vi "Change Tag Output.vi"(6 "Variant":variant, 8 "error in":errorcluster, 9 "old values":string[][](array[string]), 10 "object ref in":T1, 11 "Cluster":T2) -> (0 "error out":errorcluster)   [LabVIEW 2013, in "Shared Memory Editor Node.lvclass"]
doc: "Copyright 2016 National Instruments Corporation\n\nLicensed under the Apache License, Version 2.0 (the \"License\"); you may not use this file except in compliance with the License. You may obtain a copy of the License at http://www.apache.org/licenses/LICENSE-2.0\nUnless required by applicable law or agreed to in writing, software distributed under the License is distributed on an \"AS IS\" BASIS, WITHOUT WARRANTIES OR CONDITIONS OF ANY KIND, either express or implied. See the License for the specific language governing permissions and limitations under the License."
uses:
  Shared Memory Editor Node.lvclass
  <vilib>/NI/DCAF Table API/Table Manager/Cell Change.ctl
  <vilib>/NI/DCAF Table API/Table Manager/object ref.ctl
  <vilib>/NI/DCAF/Tag Editor Core/Configuration Editor/Classes/Engine Parent/Engine Parent Editor Node.lvclass
  <vilib>/NI/DCAF/Tag Editor Core/Configuration Editor/Classes/Module editor node/module editor node.lvclass
  <vilib>/NI/Tag Bus Module Framework/channel/TBM channel.lvclass
  <vilib>/NI/Tag Bus/tag/tag descriptor.lvclass/tag descriptor.ctl
  module/configuration/Shared Memory Configuration.lvclass
  module/configuration/Shared Memory Configuration.lvclass/Shared Memory Configuration.ctl
  <vilib>/NI/Tag Bus/tag/tag descriptor.lvclass
  <vilib>/NI/DCAF Table API/Table Manager.lvlib
  <vilib>/NI/DCAF Table API/Table Manager/Table Manager.lvclass
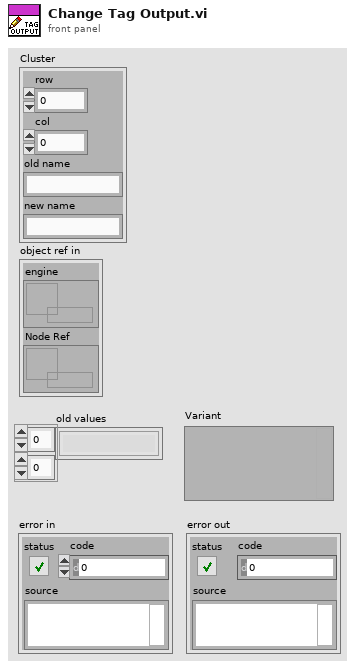
[diagram p1: front panel]
types:
  T1 = typedef "Table Manager.lvlib/Table Manager.lvclass/object ref.ctl" = cluster{"engine":refnum<data-value>, "Node Ref":refnum<data-value>}
  T2 = typedef "Table Manager.lvlib/Cell Change.ctl" = cluster{"row":i32, "col":i32, "old name":string, "new name":string}
  T3 = typedef "Shared Memory Configuration.lvclass/line configuration.ctl" = cluster{"name":string, "data type":T4, "channel":refnum<class "TBM channel.lvclass">}
  T4 = typedef "tag bus.lvlib/tag descriptor.lvclass/Data Type.ctl" = enum16{"Double", "Single", "I64", "I32", "I16", "I8", "U64", "U32", "U16", "U8", "Boolean", "String", "Array of Double", "Array of Single", "Array of I64", "Array of I32", "Array of I16", "Array of I8", "Array of U64", "Array of U32", "Array of U16", "Array of U8", "Array of Boolean", "Array of String"}
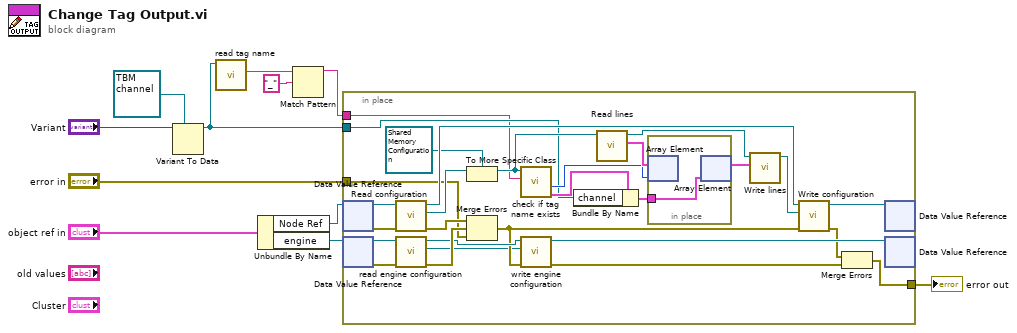
[diagram p0: block diagram]
diagram:
  n1 = Variant To Data(type=refnum<class "TBM channel.lvclass"> refnum ("output"), Variant="Variant") -> (data=w4:refnum<class "TBM channel.lvclass">)  [unwired: 1 in, 1 out]
  n2 = call <vilib>:"read tag name.vi"("system tag in"=w4) -> ("name"=w3:string)  [unwired: 8 in, 2 out]
  n3 = Unbundle By Name("object ref in") -> ("Node Ref"=w7:refnum<data-value>, "engine"=w6:refnum<data-value>)
  n4 = Match Pattern(string=w3, regular expression="_") -> (before substring=w1:string)  [unwired: 1 in, 3 out]
  n5 = in-place {
    in-place-border: [w31] -> w11
    in-place-border: "error in" -> [w23]
    in-place-border: w4 -> [w14]
    in-place-border: w1 -> [w13]
    n6 = in-place-dvr #1(w7) -> (w28:refnum<class "module editor node.lvclass">, w30:errorcluster)
    n7 = in-place-dvr #2(w6) -> (w38:refnum<class "Engine Parent Editor Node.lvclass">, w39:errorcluster)
    n8 = call-dynamic "Read configuration.vi"("error in"=w30, "NISE_CEF_serializable node in"=w28) -> ("error out"=w29:errorcluster, "configuration"=w26:refnum<class "NISE_CEF_serializable configuration.lvclass">, "NISE_CEF_serializable node out"=w27:refnum<class "module editor node.lvclass">)  [unwired: 7 in]
    n9 = call <vilib>:"read engine configuration.vi"("error in"=w39, "Engine Parent Editor Node in"=w38) -> ("error out"=w35:errorcluster, "engine configuration"=w12:refnum<class "engine configuration.lvclass">, "Engine Parent Editor Node out"=w34:refnum<class "Engine Parent Editor Node.lvclass">)  [unwired: 7 in]
    n10 = To More Specific Class(target class=refnum<class "Shared Memory Configuration.lvclass"> refnum ("tag select module configuration"), reference=w26) -> (specific class reference=w22:refnum<class "Shared Memory Configuration.lvclass">)  [unwired: 1 in, 1 out]
    n11 = Merge Errors(w29, w35, w23) -> (w25:errorcluster)
    n12 = call "check if tag name exists.vi"("name to locate"=w13, "shared memory module configuration in"=w22) -> ("tag config"=w17:T3, "index"=w18:i32)  [unwired: 6 in, 2 out]
    n13 = call <vilib>:"write engine configuration.vi"("error in"=w25, "engine configuration"=w12, "Engine Parent Editor Node in"=w34) -> ("error out"=w33:errorcluster, "Engine Parent Editor Node out"=w37:refnum<class "Engine Parent Editor Node.lvclass">)  [unwired: 7 in]
    n14 = Bundle By Name(cluster=w17, "channel"=w14) -> (w16:T3)
    n15 = call "Read lines.vi"("shared memory module configuration"=w22) -> ("lines"=w21:T3[], "shared memory module configuration out"=w19:refnum<class "Shared Memory Configuration.lvclass">)  [unwired: 8 in, 1 out]
    n16 = in-place {
      in-place-border: w16 -> [w40]
      n17 = in-place-array #3(w21, w18) -> ()  [unwired: 1 out]
      n18 = in-place-array #3(w40) -> (w20:T3[])  [unwired: 1 out]
    }
    n19 = call "Write lines.vi"("lines"=w20, "shared memory module configuration"=w19) -> ("shared memory module configuration out"=w15:refnum<class "Shared Memory Configuration.lvclass">)  [unwired: 8 in, 1 out]
    n20 = call-dynamic "Write configuration.vi"("error in"=w25, "configuration"=w15, "NISE_CEF_serializable node in"=w27) -> ("error out"=w32:errorcluster, "NISE_CEF_serializable node out"=w36:refnum<class "module editor node.lvclass">)  [unwired: 7 in]
    n21 = Merge Errors(w32, w33) -> (w31:errorcluster)
    n22 = in-place-dvr #1(w36) -> ()  [unwired: 2 out]
    n23 = in-place-dvr #2(w37) -> ()  [unwired: 2 out]
  }
  "error out" <- w11
